vi "XY to Picture Point.vi"(10 "scaling info":T1={"pixels per unit"=1.0, "fit radius (units)"=1.0, "center point (pixels)"={"x"=0, "y"=0}}, 11 "xy point (units)":cluster{"x":dbl, "y":dbl}) -> (3 "xy point (pixels)":cluster{"x":i16, "y":i16})   [LabVIEW 2017, in "NI_Robotics_2D Rangefinder Picture.lvlib"]
uses:
  <vilib>/robotics/Controls/2D Rangefinder/2D Rangefinder Picture/NI_Robotics_2D Rangefinder Picture.lvlib
  <vilib>/robotics/Controls/2D Rangefinder/2D Rangefinder Picture/Scaling Info.ctl
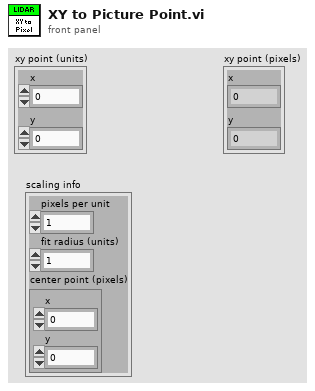
[diagram p1: front panel]
types:
  T1 = typedef "NI_Robotics_2D Rangefinder Picture.lvlib/Scaling Info.ctl" = cluster{"pixels per unit":dbl, "fit radius (units)":dbl, "center point (pixels)":cluster{"x":i16, "y":i16}}
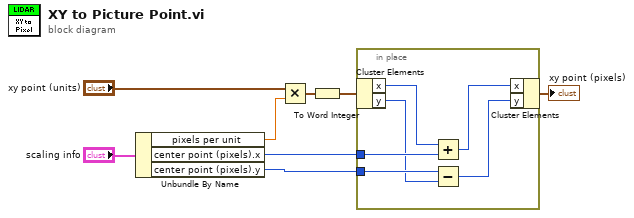
[diagram p0: block diagram]
diagram:
  n1 = Unbundle By Name("scaling info") -> ("pixels per unit"=w7:dbl, "center point (pixels).x"=w4:i16, "center point (pixels).y"=w3:i16)
  n2 = Multiply(x="xy point (units)", y=w7) -> (x*y=w5:cluster{"x":dbl, "y":dbl})
  n3 = To Word Integer(number=w5) -> (16bit integer=w2:cluster{"x":i16, "y":i16})
  n4 = in-place {
    in-place-border: w4 -> [w14]
    in-place-border: w3 -> [w13]
    n5 = in-place-cluster #1(w2) -> ("x"=w12:i16, "y"=w11:i16)
    n6 = Add(x=w12, y=w14) -> (x+y=w10:i16)
    n7 = Subtract(x=w13, y=w11) -> (x-y=w9:i16)
    n8 = in-place-cluster #1("x"=w10, "y"=w9) -> (→"xy point (pixels)":cluster{"x":i16, "y":i16})
  }
